vi "Load Signal Bank 1.0.3.vi"(4 "error in (no error)":errorcluster, 5 "Input array":dbl[][](array[numeric])=array10000x1[10000 elements] format="%.2f", 6 "CCA":cluster{"channel":string, "channel on":bool}[](array[cluster])=[{"channel"="0", "channel on"=TRUE}, {"channel"="1", "channel on"=TRUE}, {"channel"="2", "channel on"=TRUE}, {"channel"="3", "channel on"=TRUE}, {"channel"="4", "channel on"=FALSE}, {"channel"="5", "channel on"=FALSE}, {"channel"="6", "channel on"=FALSE}, {"channel"="7", "channel on"=FALSE}], 7 "timeout (ms)":i32=5000) -> (0 "error out":errorcluster={"status"=FALSE, "code"=0, "source"="."})   [LabVIEW 2015]
uses:
  DAQ Engine VIs/PXI Globals.vi
panel:
  in  "Action":enum16{"Add", "Replace ID", "Read ID", "Clear"}(ring)
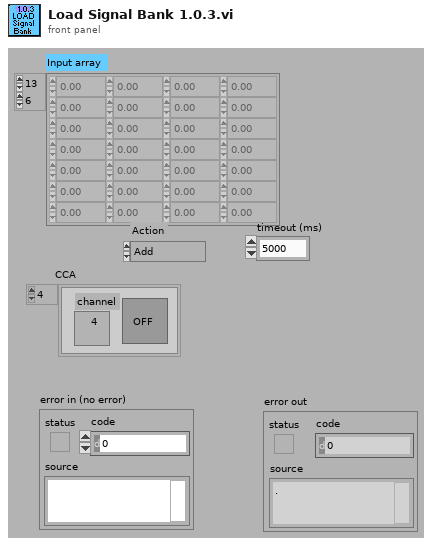
[diagram p1: front panel]
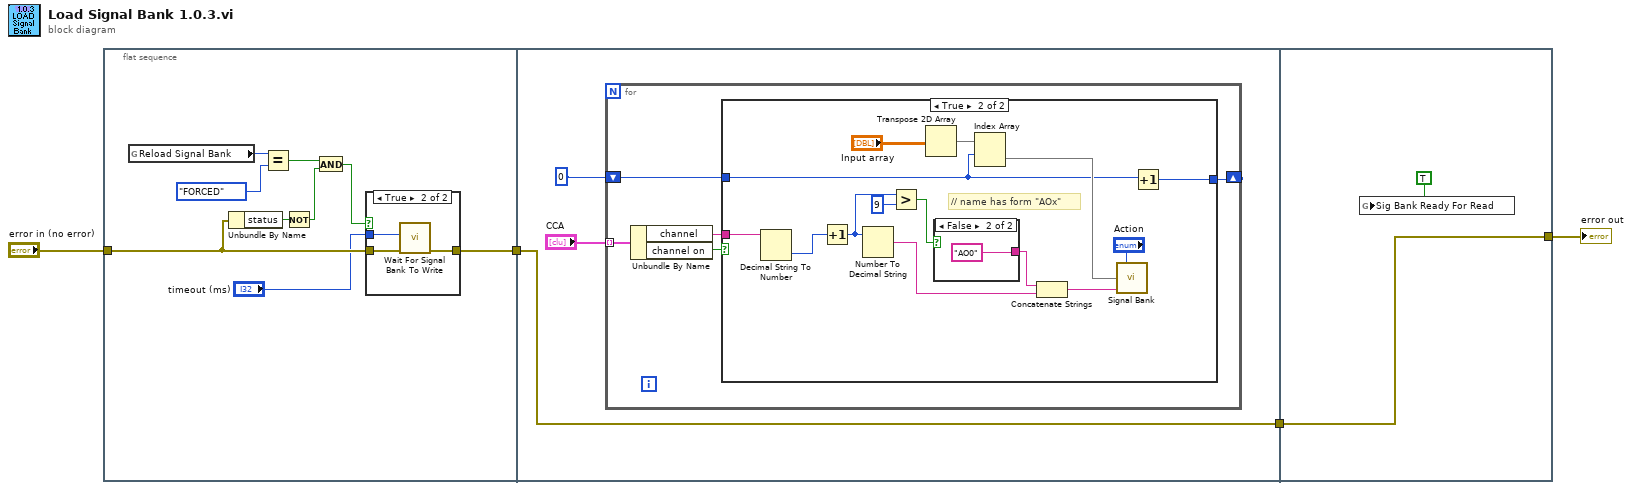
[diagram p0: block diagram]
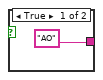
[diagram p4: hidden frame]
diagram:
  n1 = flat-sequence {
    tunnel: "error in (no error)" -> [w6]
    tunnel: [w13] -> w3
    tunnel: w3 -> [w18]
    tunnel: [w18] -> w2
    tunnel: [w43] -> w1
    tunnel: w2 -> [w43]
    frame #0 {
      n2 = global read "PXI Globals.vi" "Reload Signal Bank"() -> (w8:enum32{"OFF", "ENABLED", "FORCED"})
      n3 = Unbundle By Name(w6) -> ("status"=w10:bool)
      n4 = Equal?(x=w8, y=enum16{"OFF", "ENABLED", "FORCED"}."FORCED") -> (x = y?=w12:bool)
      n5 = Not(x=w10) -> (.not. x?=w11:bool)
      n6 = And(x=w12, y=w11) -> (x .and. y?=w7:bool)
      n7 = case shown="True" w7 {
        tunnel: w6 -> [w14 w17]
        tunnel: [w14 w16] -> w13
        tunnel: "timeout (ms)" -> [_ w15]
        frame False {
        }
        frame True {
          n8 = call "Wait For Signal Bank To Write.vi"("error in (no error)"=w17, "timeout (ms)"=w15) -> ("error out"=w16:errorcluster)  [unwired: 8 in, 1 out]
        }
      }
    }
    frame #1 {
      n9 = for {
        tunnel: "CCA" -> [w25] mode=indexing
        shift-right: [w21] -> _
        shift-left: 0 -> [w22]
        n10 = Unbundle By Name(w25) -> ("channel"=w24:string, "channel on"=w23:bool)
        n11 = case shown="True" w23 {
          tunnel: w24 -> [_ w32]
          tunnel: w22 -> [w26 w35]
          tunnel: [w26 w36] -> w21
          frame False {
          }
          frame True {
            # "// name has form \"AOx\""
            n12 = Decimal String To Number(string=w32) -> (number=w31:i32)  [unwired: 2 in, 1 out]
            n13 = Increment(x=w31) -> (x+1=w28:i32)
            n14 = Number To Decimal String(number=w28) -> (decimal integer string=w33:string)  [unwired: 1 in]
            n15 = Greater?(x=w28, y=9) -> (0:w29:bool)
            n16 = Transpose 2D Array(2D array="Input array") -> (transposed array=w34:dbl[][])
            n17 = case shown="False" w29 {
              tunnel: ["AO" "AO0"] -> w27
              frame True {
              }
              frame False {
              }
            }
            n18 = Index Array(array=w34, index (row)=w35) -> (element=w37:dbl[])  [unwired: 1 in]
            n19 = Concatenate Strings(w27, w33) -> (w40:string)
            n20 = call "Signal Bank.vi"("Action"="Action", "1D Data In"=w37, "ID"=w40) -> ()  [unwired: 11 in, 2 out]
            n21 = Increment(x=w35) -> (x+1=w36:i32)
          }
        }
      }
    }
    frame #2 {
      n22 = global write "PXI Globals.vi" "Sig Bank Ready For Read"(TRUE) -> ()
    }
  }
  "error out" <- w1
